vi "显示UI.vi"() -> ()   [LabVIEW 2016, in "国弘多参数.lvlib"]
uses:
  <vilib>/Utility/miscctls.llb/LVPointTypeDef.ctl
  <vilib>/Utility/config.llb/NI_LVConfig.lvlib
panel:
  out "运行状态":u16(ring) items=["空闲", "水样测试", "标样核查"]
  in  "叶绿素a校准":bool
  in  "停止":bool
  in  "标样核查":bool
  in  "水样测试":bool
  in  "关闭":bool
  in  "open MB":bool
  in  "设置":bool
  in  "水温校准":bool
  in  "浊度校准":bool
  in  "溶解氧校准":bool
  in  "电导率校准":bool
  in  "pH校准":bool
  in  "探头校正返回":bool
  in  "探头校正":bool
  in  "浊度参数查询":bool
  in  "溶解氧参数查询":bool
  in  "电导率参数查询":bool
  in  "pH参数查询":bool
  out "检测值":T1
  in  "返回":bool
  in  "参数查询":bool
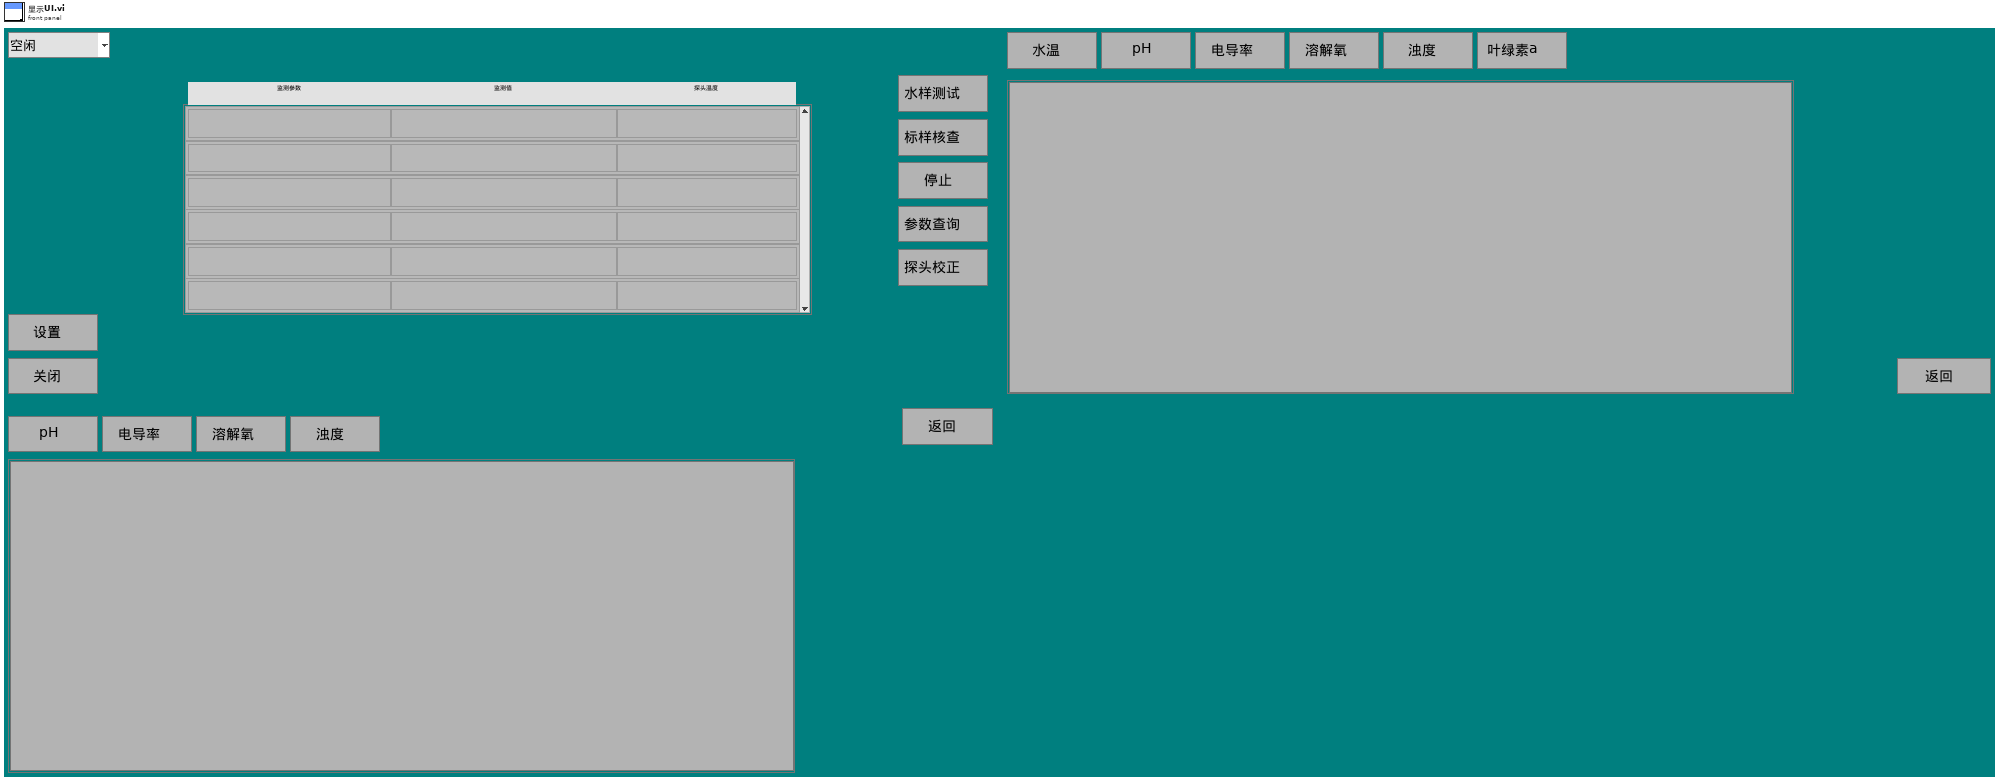
[diagram p1: front panel]
types:
  T1 = typedef "国弘多参数.lvlib/检测值.ctl" = cluster{"监测参数1":string, "浓度1":string, "探头温度1":string}[]
  T2 = typedef "LVPointTypeDef.ctl" = cluster{"Horizontal":i16, "Vertical":i16}
  T3 = cluster{"电极状态标志":u16, "电极型号标志":u16, "溶解氧测量值":sgl, "温度测量值":sgl, "溶解氧饱和度值":sgl, "盐度补偿值":sgl, "大气压补偿值":sgl, "溶解氧偏移修正值":sgl, "温度偏移修正值":sgl, "手动温度补偿值":sgl, "溶解氧电极零点":sgl, "溶解氧电极斜率":sgl, "第1点标准值记录":sgl, "第1点信号值记录":sgl, "第1点温度值记录":sgl, "第2点标准值记录":sgl, "第2点信号值记录":sgl, "第2点温度值记录":sgl, "命令滤波设定":u16, "温度模式":enum16{"ATC", "MTC"}, "生产批次":u16, "电极序号":u16, "串口地址":u16, "串口波特率":enum16{"9600", "19200", "115200"}, "串口校验位":enum16{"NONE", "ODD", "EVEN"}, "串口停止位":enum16{"1bit", "2bit"}, "第一点标准值":sgl, "第二点标准值":sgl}
  T4 = cluster{"电极状态标志":u16, "电极型号标志":u16, "酸碱度测量值":sgl, "温度测量值":sgl, "酸碱度信号值":sgl, "温度信号值":sgl, "酸碱度偏移修正值":sgl, "温度偏移修正值":sgl, "手动温度补偿值":sgl, "酸碱度电极零点":sgl, "酸碱度电极斜率":sgl, "第1点标准值记录":sgl, "第1点信号值记录":sgl, "第1点温度值记录":sgl, "第2点标准值记录":sgl, "第2点信号值记录":sgl, "第2点温度值记录":sgl, "命令滤波设定":u16, "温度模式":enum16{"ATC", "MTC"}, "生产批次":u16, "电极序号":u16, "串口地址":u16, "串口波特率":enum16{"9600", "19200", "115200"}, "串口校验位":enum16{"NONE", "ODD", "EVEN"}, "串口停止位":enum16{"1bit", "2bit"}, "第一点标准值":sgl, "第二点标准值":sgl}
  T5 = cluster{"电极状态标志":u16, "电极型号标志":u16, "浊度测量值":sgl, "温度测量值":sgl, "浊度信号值":sgl, "浊度偏移修正值":sgl, "温度偏移修正值":sgl, "手动温度补偿值":sgl, "浊度电极零点":sgl, "浊度电极斜率":sgl, "第1点标准值记录":sgl, "第1点信号值记录":sgl, "第1点温度值记录":sgl, "第2点标准值记录":sgl, "第2点信号值记录":sgl, "第2点温度值记录":sgl, "命令滤波设定":u16, "温度模式":enum16{"ATC", "MTC"}, "生产批次":u16, "电极序号":u16, "串口地址":u16, "串口波特率":enum16{"9600", "19200", "115200"}, "串口校验位":enum16{"NONE", "ODD", "EVEN"}, "串口停止位":enum16{"1bit", "2bit"}, "第一点标准值":sgl, "第二点标准值":sgl}
  T6 = cluster{"电极状态标志":u16, "电极型号标志":u16, "电导率测量值":sgl, "温度测量值":sgl, "电导率信号值":sgl, "温度信号值":sgl, "温度补偿系数":sgl, "电导率偏移修正值":sgl, "温度偏移修正值":sgl, "手动温度补偿值":sgl, "电导率电极零点":sgl, "电导率电极斜率":sgl, "命令滤波设定":u16, "温度模式":enum16{"ATC", "MTC"}, "生产批次":u16, "电极序号":u16, "串口地址":u16, "串口波特率":enum16{"9600", "19200", "115200"}, "串口校验位":enum16{"NONE", "ODD", "EVEN"}, "串口停止位":enum16{"1bit", "2bit"}, "第一点标准值":sgl, "第二点标准值":sgl}
  T7 = cluster{"监测参数1":string, "浓度1":string, "探头温度1":string}[]
  T8 = cluster{"CH":u16, "监测值":dbl, "监测信号值":dbl, "温度偏移修正值":sgl}
  T9 = typedef "NI_LVConfig.lvlib/Config Data RefNum.ctl" = refnum<k1>
  T10 = cluster{"baud rate (bps)":u32, "stop bits":u16, "parity":u16, "flow control":u16, "timeout":u32, "retries":i32}
  T11 = enum32{"Bad", "Idle", "Run top level", "Running"}
  T12 = cluster{"数据保存间隔":dbl, "水温标样值":dbl, "pH标样值":dbl, "溶解氧标样值":dbl, "电导率标样值":dbl, "浊度标样值":dbl}
  T13 = cluster{"Temp":bool, "pH":bool, "DO":bool, "Cond":bool, "Turb":bool, "叶绿素a启用":bool}
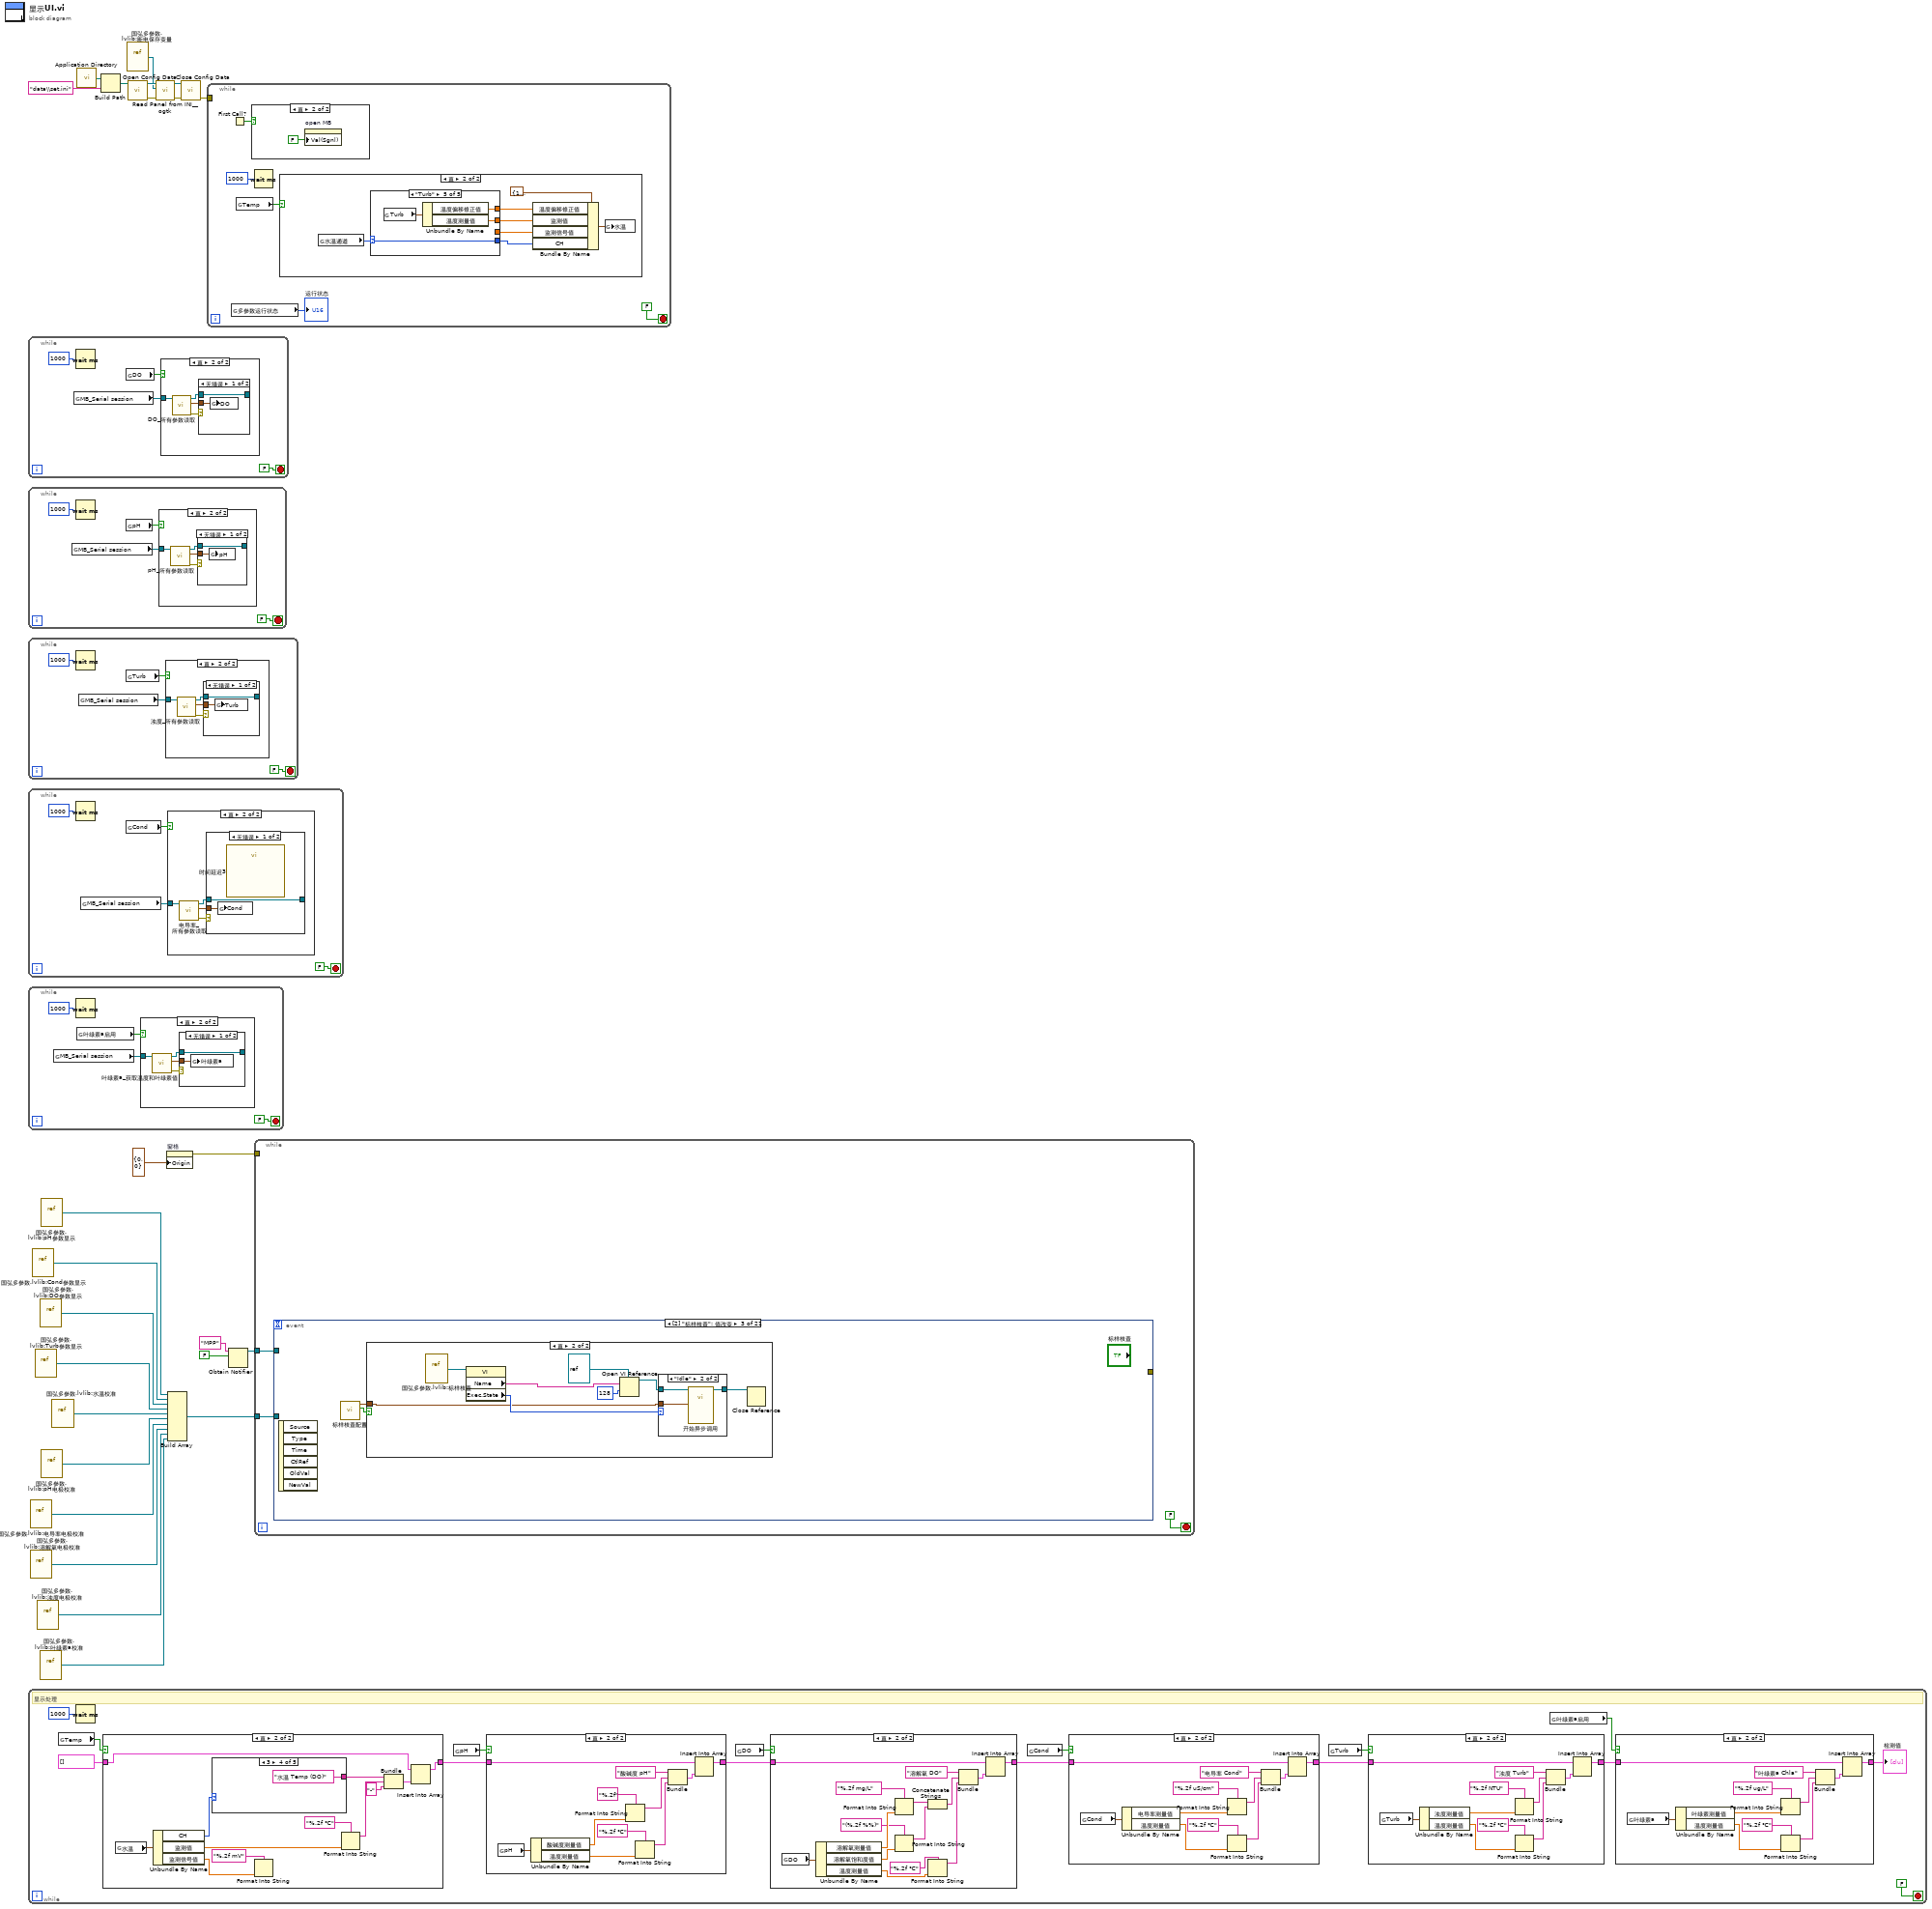
[diagram p0: block diagram]
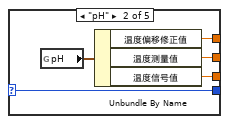
[diagram p14: hidden frame]
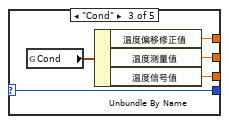
[diagram p15: hidden frame]
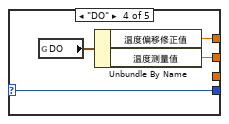
[diagram p16: hidden frame]
diagram:
  n1 = while {
    stop <- FALSE stop-if-true
    n2 = global read "过程全局变量.vi" "MB_Serial session"() -> (w26:refnum<class "MB_Master_Serial.lvclass">)
    n3 = Wait (ms)(milliseconds to wait=u32 1000 ("等待时间（毫秒）")) -> ()  [unwired: 1 out]
    n4 = global read "断电保存变量.vi" "DO"() -> (w27:bool)
    n5 = case shown="真" w27 {
      tunnel: w26 -> [_ w30]
      frame False {
      }
      frame True {
        n6 = call "DO_所有参数读取.vi"("MB_Serial session in"=w30) -> ("error out"=w32:errorcluster, "输出值"=w33:T3, "MB_Serial session out"=w31:refnum<class "MB_Master_Serial.lvclass">)  [unwired: 8 in]
        n7 = case shown="无错误" w32 {
          tunnel: w33 -> [w35 _]
          tunnel: w31 -> [w34 w36]
          tunnel: [w34 w36] -> _
          frame No Error {
            n8 = global write "过程全局变量.vi" "DO"(w35) -> ()
          }
          frame Error {
          }
        }
      }
    }
  }
  n9 = while {
    stop <- FALSE stop-if-true
    n10 = global read "过程全局变量.vi" "MB_Serial session"() -> (w38:refnum<class "MB_Master_Serial.lvclass">)
    n11 = Wait (ms)(milliseconds to wait=u32 1000 ("等待时间（毫秒）")) -> ()  [unwired: 1 out]
    n12 = global read "断电保存变量.vi" "pH"() -> (w39:bool)
    n13 = case shown="真" w39 {
      tunnel: w38 -> [_ w41]
      frame False {
      }
      frame True {
        n14 = call "pH_所有参数读取.vi"("MB_Serial session in"=w41) -> ("error out"=w43:errorcluster, "输出值"=w44:T4, "MB_Serial session out"=w42:refnum<class "MB_Master_Serial.lvclass">)  [unwired: 8 in]
        n15 = case shown="无错误" w43 {
          tunnel: w44 -> [w46 _]
          tunnel: w42 -> [w45 w47]
          tunnel: [w45 w47] -> _
          frame No Error {
            n16 = global write "过程全局变量.vi" "pH"(w46) -> ()
          }
          frame Error {
          }
        }
      }
    }
  }
  n17 = while {
    stop <- FALSE stop-if-true
    n18 = Wait (ms)(milliseconds to wait=u32 1000 ("等待时间（毫秒）")) -> ()  [unwired: 1 out]
    n19 = global read "过程全局变量.vi" "MB_Serial session"() -> (w49:refnum<class "MB_Master_Serial.lvclass">)
    n20 = global read "断电保存变量.vi" "Turb"() -> (w50:bool)
    n21 = case shown="真" w50 {
      tunnel: w49 -> [_ w52]
      frame False {
      }
      frame True {
        n22 = call "浊度_所有参数读取.vi"("MB_Serial session in"=w52) -> ("error out"=w54:errorcluster, "输出值"=w55:T5, "MB_Serial session out"=w53:refnum<class "MB_Master_Serial.lvclass">)  [unwired: 8 in]
        n23 = case shown="无错误" w54 {
          tunnel: w55 -> [w57 _]
          tunnel: w53 -> [w56 w58]
          tunnel: [w56 w58] -> _
          frame No Error {
            n24 = global write "过程全局变量.vi" "Turb"(w57) -> ()
          }
          frame Error {
          }
        }
      }
    }
  }
  n25 = while {
    stop <- FALSE stop-if-true
    n26 = Wait (ms)(milliseconds to wait=u32 1000 ("等待时间（毫秒）")) -> ()  [unwired: 1 out]
    n27 = global read "过程全局变量.vi" "MB_Serial session"() -> (w60:refnum<class "MB_Master_Serial.lvclass">)
    n28 = global read "断电保存变量.vi" "Cond"() -> (w61:bool)
    n29 = case shown="真" w61 {
      tunnel: w60 -> [_ w63]
      frame False {
      }
      frame True {
        n30 = call "电导率_所有参数读取.vi"("MB_Serial session in"=w63) -> ("error out"=w65:errorcluster, "输出值"=w66:T6, "MB_Serial session out"=w64:refnum<class "MB_Master_Serial.lvclass">)  [unwired: 8 in]
        n31 = case shown="无错误" w65 {
          tunnel: w66 -> [w68 _]
          tunnel: [w67 w69] -> _
          tunnel: w64 -> [w67 w69]
          frame No Error {
            n32 = global write "过程全局变量.vi" "Cond"(w68) -> ()
            n33 = call "时间延迟3"() -> ()  [unwired: 11 in, 1 out]
          }
          frame Error {
          }
        }
      }
    }
  }
  n34 = while {
    stop <- FALSE stop-if-true
    n35 = global read "过程全局变量.vi" "MB_Serial session"() -> (w72:refnum<class "MB_Master_Serial.lvclass">)
    n36 = Wait (ms)(milliseconds to wait=u32 1000 ("等待时间（毫秒）")) -> ()  [unwired: 1 out]
    n37 = global read "断电保存变量.vi" "叶绿素a启用"() -> (w71:bool)
    n38 = case shown="真" w71 {
      tunnel: w72 -> [_ w74]
      frame False {
      }
      frame True {
        n39 = call "叶绿素a_获取温度和叶绿素值.vi"("MB_Serial session in"=w74) -> ("error out"=w76:errorcluster, "输出值"=w77:cluster{"温度测量值":sgl, "叶绿素测量值":sgl, "错误标志":u16}, "MB_Serial session out"=w75:refnum<class "MB_Master_Serial.lvclass">)  [unwired: 8 in]
        n40 = case shown="无错误" w76 {
          tunnel: w77 -> [w79 _]
          tunnel: w75 -> [w78 w80]
          tunnel: [w78 w80] -> _
          frame No Error {
            n41 = global write "过程全局变量.vi" "叶绿素a"(w79) -> ()
          }
          frame Error {
          }
        }
      }
    }
  }
  n42 = while {
    stop <- FALSE stop-if-true
    # "显示处理"
    n43 = global read "断电保存变量.vi" "Temp"() -> (w93:bool)
    n44 = Wait (ms)(milliseconds to wait=u32 1000 ("等待时间（毫秒）")) -> ()  [unwired: 1 out]
    n45 = case shown="真" w93 {
      tunnel: [w160 w161] -> w90
      tunnel: T7 [] ("数组") -> [w160 w162]
      frame False {
      }
      frame True {
        n46 = global read "过程全局变量.vi" "水温"() -> (w172:T8)
        n47 = Unbundle By Name(w172) -> ("CH"=w167:u16, "监测值"=w170:dbl, "监测信号值"=w168:dbl)
        n48 = case shown="3" w167 {
          tunnel: ["水温 Temp" ("监测参数1") "水温 Temp (pH)" ("监测参数1") "水温 Temp (Cond)" ("监测参数1") "水温 Temp (DO)" ("监测参数1") "水温 Temp (Turb)" ("监测参数1")] -> w166
          frame 0, Default {
          }
          frame 1 {
          }
          frame 2 {
          }
          frame 3 {
          }
          frame 4 {
          }
        }
        n49 = Format Into String(format string="%.2f mV" ("格式字符串"), w168) -> ()  [unwired: 2 in, 2 out]
        n50 = Format Into String(format string="%.2f ℃" ("格式字符串"), w170) -> (resulting string=w165:string)  [unwired: 2 in, 1 out]
        n51 = Bundle("监测参数1"=w166, w165, "探头温度1"="-") -> (w163:cluster{"监测参数1":string, string, "探头温度1":string})  [unwired: 1 in]
        n52 = Insert Into Array(array=w162, new element=w163) -> (w161:T7)  [unwired: 1 in]
      }
    }
    n53 = global read "断电保存变量.vi" "pH"() -> (w91:bool)
    n54 = case shown="真" w91 {
      tunnel: [w148 w149] -> w88
      tunnel: w90 -> [w148 w151]
      frame False {
      }
      frame True {
        n55 = global read "过程全局变量.vi" "pH"() -> (w159:T4)
        n56 = Unbundle By Name(w159) -> ("酸碱度测量值"=w158:sgl, "温度测量值"=w156:sgl)
        n57 = Format Into String(format string="%.2f" ("格式字符串"), w158) -> (resulting string=w152:string)  [unwired: 2 in, 1 out]
        n58 = Format Into String(format string="%.2f ℃" ("格式字符串"), w156) -> (resulting string=w154:string)  [unwired: 2 in, 1 out]
        n59 = Bundle("监测参数2"="酸碱度 pH", w152, w154) -> (w150:cluster{"监测参数2":string, string, string})  [unwired: 1 in]
        n60 = Insert Into Array(array=w151, new element=w150) -> (w149:T7)  [unwired: 1 in]
      }
    }
    n61 = global read "断电保存变量.vi" "DO"() -> (w89:bool)
    n62 = case shown="真" w89 {
      tunnel: [w132 w133] -> w85
      tunnel: w88 -> [w132 w134]
      frame False {
      }
      frame True {
        n63 = global read "过程全局变量.vi" "DO"() -> (w143:T3)
        n64 = Unbundle By Name(w143) -> ("溶解氧测量值"=w144:sgl, "溶解氧饱和度值"=w141:sgl, "温度测量值"=w146:sgl)
        n65 = Format Into String(format string="%.2f mg/L" ("格式字符串"), w144) -> (resulting string=w140:string)  [unwired: 2 in, 1 out]
        n66 = Format Into String(format string="(%.2f %%)" ("格式字符串"), w141) -> (resulting string=w139:string)  [unwired: 2 in, 1 out]
        n67 = Concatenate Strings(w140, w139) -> (w138:string)
        n68 = Format Into String(format string="%.2f ℃" ("格式字符串"), w146) -> (resulting string=w136:string)  [unwired: 2 in, 1 out]
        n69 = Bundle("监测参数2"="溶解氧 DO", w138, w136) -> (w135:cluster{"监测参数2":string, string, string})  [unwired: 1 in]
        n70 = Insert Into Array(array=w134, new element=w135) -> (w133:T7)  [unwired: 1 in]
      }
    }
    n71 = global read "断电保存变量.vi" "Cond"() -> (w87:bool)
    n72 = case shown="真" w87 {
      tunnel: w85 -> [w120 w123]
      tunnel: [w120 w121] -> w84
      frame False {
      }
      frame True {
        n73 = global read "过程全局变量.vi" "Cond"() -> (w131:T6)
        n74 = Unbundle By Name(w131) -> ("电导率测量值"=w130:sgl, "温度测量值"=w128:sgl)
        n75 = Format Into String(format string="%.2f uS/cm" ("格式字符串"), w130) -> (resulting string=w124:string)  [unwired: 2 in, 1 out]
        n76 = Format Into String(format string="%.2f ℃" ("格式字符串"), w128) -> (resulting string=w125:string)  [unwired: 2 in, 1 out]
        n77 = Bundle("监测参数2"="电导率 Cond", w124, w125) -> (w122:cluster{"监测参数2":string, string, string})  [unwired: 1 in]
        n78 = Insert Into Array(array=w123, new element=w122) -> (w121:T7)  [unwired: 1 in]
      }
    }
    n79 = global read "断电保存变量.vi" "Turb"() -> (w86:bool)
    n80 = case shown="真" w86 {
      tunnel: w84 -> [w108 w111]
      tunnel: [w108 w109] -> w83
      frame False {
      }
      frame True {
        n81 = global read "过程全局变量.vi" "Turb"() -> (w115:T5)
        n82 = Unbundle By Name(w115) -> ("浊度测量值"=w116:sgl, "温度测量值"=w118:sgl)
        n83 = Format Into String(format string="%.2f NTU" ("格式字符串"), w116) -> (resulting string=w113:string)  [unwired: 2 in, 1 out]
        n84 = Format Into String(format string="%.2f ℃" ("格式字符串"), w118) -> (resulting string=w114:string)  [unwired: 2 in, 1 out]
        n85 = Bundle("监测参数2"="浊度 Turb", w113, w114) -> (w110:cluster{"监测参数2":string, string, string})  [unwired: 1 in]
        n86 = Insert Into Array(array=w111, new element=w110) -> (w109:T7)  [unwired: 1 in]
      }
    }
    n87 = global read "断电保存变量.vi" "叶绿素a启用"() -> (w81:bool)
    n88 = case shown="真" w81 {
      tunnel: w83 -> [w96 w99]
      tunnel: [w96 w97] -> w82
      frame False {
      }
      frame True {
        n89 = global read "过程全局变量.vi" "叶绿素a"() -> (w103:cluster{"温度测量值":sgl, "叶绿素测量值":sgl, "错误标志":u16})
        n90 = Unbundle By Name(w103) -> ("叶绿素测量值"=w104:sgl, "温度测量值"=w106:sgl)
        n91 = Format Into String(format string="%.2f ug/L" ("格式字符串"), w104) -> (resulting string=w101:string)  [unwired: 2 in, 1 out]
        n92 = Format Into String(format string="%.2f ℃" ("格式字符串"), w106) -> (resulting string=w102:string)  [unwired: 2 in, 1 out]
        n93 = Bundle("监测参数2"="叶绿素a Chla", w101, w102) -> (w98:cluster{"监测参数2":string, string, string})  [unwired: 1 in]
        n94 = Insert Into Array(array=w99, new element=w98) -> (w97:T7)  [unwired: 1 in]
      }
    }
    "检测值" <- w82
  }
  n95 = vi-ref "国弘多参数.lvlib:电导率电极校准.vi"() -> (w16:refnum<vi>)
  n96 = vi-ref "国弘多参数.lvlib:溶解氧电极校准.vi"() -> (w15:refnum<vi>)
  n97 = vi-ref "国弘多参数.lvlib:Cond参数显示.vi"() -> (w22:refnum<vi>)
  n98 = vi-ref "国弘多参数.lvlib:Turb参数显示.vi"() -> (w20:refnum<vi>)
  n99 = vi-ref "国弘多参数.lvlib:浊度电极校准.vi"() -> (w14:refnum<vi>)
  n100 = vi-ref "国弘多参数.lvlib:DO参数显示.vi"() -> (w21:refnum<vi>)
  n101 = vi-ref "国弘多参数.lvlib:叶绿素a校准.vi"() -> (w4:refnum<vi>)
  n102 = vi-ref "国弘多参数.lvlib:pH参数显示.vi"() -> (w23:refnum<vi>)
  n103 = vi-ref "国弘多参数.lvlib:pH电极校准.vi"() -> (w17:refnum<vi>)
  n104 = vi-ref "国弘多参数.lvlib:水温校准.vi"() -> (w18:refnum<vi>)
  n105 = call <vilib>:"Application Directory.vi"() -> ("Application Directory"=w9:path)
  n106 = Build Path(base path=w9, name or relative path="data\\set.ini" ("名称或相对路径")) -> (appended path=w8:path)
  n107 = vi-ref "国弘多参数.lvlib:断电保存变量.vi"() -> (w6:refnum<vi>)
  n108 = call <vilib>:"Open Config Data.vi"("configuration file path"=w8) -> ("error out"=w12:errorcluster, "refnum"=w13:T9)  [unwired: 8 in, 1 out]
  n109 = call <userlib>:"Read Panel from INI__ogtk.vi"("error in (no error)"=w12, "VI ref"=w6, "refnum"=w13) -> ("error out"=w10:errorcluster, "refnum out"=w11:T9)  [unwired: 7 in]
  n110 = property on="窗格" class="Pane"("Origin"=T2 {"Horizontal"=0, "Vertical"=0} ("原点")) -> (error out=w25:errorcluster)  [unwired: 2 in, 1 out]
  n111 = Build Array(w23, w22, w21, w20, w18, w17, w16, w15, w14, w4) -> (w19:refnum<vi>[])
  n112 = call <vilib>:"Close Config Data.vi"("error in (no error)"=w10, "refnum"=w11) -> ("error out"=w5:errorcluster)  [unwired: 8 in, 1 out]
  n113 = while {
    tunnel: w5 -> [_]
    stop <- FALSE stop-if-true
    n114 = First Call?() -> (First Call?: T/F=w180:bool)
    n115 = global read "过程全局变量.vi" "多参数运行状态"() -> (→"运行状态":u16)
    n116 = global read "断电保存变量.vi" "Temp"() -> (w179:bool)
    n117 = case shown="真" w180 {
      frame False {
      }
      frame True {
        n118 = property on="open MB" class="Bool (严格)"("Val(Sgnl)"=FALSE ("值(信号)")) -> ()  [unwired: 2 in, 2 out]
      }
    }
    n119 = Wait (ms)(milliseconds to wait=u32 1000 ("等待时间（毫秒）")) -> ()  [unwired: 1 out]
    n120 = case shown="真" w179 {
      frame False {
      }
      frame True {
        n121 = global read "断电保存变量.vi" "水温通道"() -> (w189:enum16{"NULL", "pH", "Cond", "DO", "Turb"})
        n122 = case shown="\"Turb\"" w189 {
          selector: w189 -> [w190 w195 w200 w204 w208]
          tunnel: [w190 w195 w200 w204 w208] -> w188
          tunnel: [_ w193 w198 w202 w206] -> w187
          tunnel: [_ w192 w197 _ _] -> w186
          tunnel: [_ w191 w196 w201 w205] -> w183
          frame "NULL", Default {
          }
          frame "pH" {
            n123 = global read "过程全局变量.vi" "pH"() -> (w194:T4)
            n124 = Unbundle By Name(w194) -> ("温度偏移修正值"=w191:sgl, "温度测量值"=w193:sgl, "温度信号值"=w192:sgl)
          }
          frame "Cond" {
            n125 = global read "过程全局变量.vi" "Cond"() -> (w199:T6)
            n126 = Unbundle By Name(w199) -> ("温度偏移修正值"=w196:sgl, "温度测量值"=w198:sgl, "温度信号值"=w197:sgl)
          }
          frame "DO" {
            n127 = global read "过程全局变量.vi" "DO"() -> (w203:T3)
            n128 = Unbundle By Name(w203) -> ("温度偏移修正值"=w201:sgl, "温度测量值"=w202:sgl)
          }
          frame "Turb" {
            n129 = global read "过程全局变量.vi" "Turb"() -> (w207:T5)
            n130 = Unbundle By Name(w207) -> ("温度偏移修正值"=w205:sgl, "温度测量值"=w206:sgl)
          }
        }
        n131 = Bundle By Name(cluster=T8 {"CH"=1, "监测值"=0.0, "监测信号值"=0.0, "温度偏移修正值"=0.0} ("水温"), "温度偏移修正值"=w183, "监测值"=w187, "监测信号值"=w186, "CH"=w188) -> (w185:T8)
        n132 = global write "过程全局变量.vi" "水温"(w185) -> ()
      }
    }
  }
  n133 = Obtain Notifier(name (unnamed)="MPP" ("名称（未命名）"), notification data type=FALSE) -> (notifier out=w1:refnum<notifier>)  [unwired: 2 in, 2 out]
  n134 = while {
    tunnel: w25 -> [_]
    tunnel: w19 -> [w211]
    tunnel: w1 -> [w210]
    stop <- FALSE stop-if-true
    n135 = event shown="[2] \"标样核查\": 值改变" {
      selector: _ -> [_ _ _ _ _ _ _ _ _ _ _ _ _ _ _ _ _ _ _ _ _]
      dyn-events: _ -> [_ _ _ _ _ _ _ _ _ _ _ _ _ _ _ _ _ _ _ _ _]
      timeout: _ -> [_ _ _ _ _ _ _ _ _ _ _ _ _ _ _ _ _ _ _ _ _]
      tunnel: w211 -> [_ _ _ _ _ _ _ w275 w287 w299 w307 w318 w330 w342 w354 w366 w378 w390 w402 w414 w426]
      tunnel: [_ _ _ _ _ w247 _ _ _ _ _ _ _ _ _ _ _ _ _ _ _] -> _
      tunnel: w210 -> [_ _ _ w244 _ _ _ _ _ _ _ _ _ _ _ _ _ _ _ _ _]
      event Timeout {
        n136 = event-data() -> ()  [unwired: 1 in, 3 out]
      }
      event "水样测试": Value Change {
        n137 = event-data() -> ()  [unwired: 1 in, 6 out]
        n138 = call "水样测试配置.vi"() -> ("确认输出"=w214:bool, "水样测定时间输出"=w213:dbl)  [unwired: 10 in]
        n139 = case shown="真" w214 {
          tunnel: w213 -> [_ w217]
          frame False {
          }
          frame True {
            n140 = vi-ref "国弘多参数.lvlib:水样测试.vi"() -> (w218:refnum<vi>)
            n141 = property class="VI"(reference=w218) -> ("Name"=w222:string, "Exec.State"=w220:T11)  [unwired: 1 in, 2 out]
            n142 = Open VI Reference(type specifier VI Refnum (for type only)=refnum<vi> refnum, vi path=w222, options=128 ("选项")) -> (vi reference=w223:refnum<vi>)  [unwired: 3 in, 1 out]
            n143 = case shown="\"Idle\"" w220 {
              tunnel: [w224 w228] -> w219
              tunnel: w223 -> [w224 w227]
              tunnel: w217 -> [_ w226]
              tunnel: "hd" ("数据标记表") -> [_ w225]
              frame "Bad", Default {
              }
              frame "Idle" {
                n144 = call-by-ref "开始异步调用"(reference=w227, "数据标记表"=w225, "水样测试时间"=w226) -> (reference out=w228:refnum<vi>)  [unwired: 11 in, 1 out]
              }
            }
            n145 = Close Reference(reference=w219) -> ()  [unwired: 1 in, 1 out]
          }
        }
      }
      event "标样核查": Value Change {
        n146 = event-data() -> ()  [unwired: 1 in, 6 out]
        n147 = call "标样核查配置.vi"() -> ("确认输出"=w230:bool, "标样核查配置"=w229:T12)  [unwired: 10 in]
        n148 = case shown="真" w230 {
          tunnel: w229 -> [_ w231]
          frame False {
          }
          frame True {
            n149 = vi-ref "国弘多参数.lvlib:标样核查.vi"() -> (w232:refnum<vi>)
            n150 = property class="VI"(reference=w232) -> ("Name"=w237:string, "Exec.State"=w234:T11)  [unwired: 1 in, 2 out]
            n151 = Open VI Reference(type specifier VI Refnum (for type only)=refnum<vi> refnum, vi path=w237, options=128 ("选项")) -> (vi reference=w238:refnum<vi>)  [unwired: 3 in, 1 out]
            n152 = case shown="\"Idle\"" w234 {
              tunnel: [w239 w242] -> w233
              tunnel: w238 -> [w239 w241]
              tunnel: w231 -> [_ w240]
              frame "Bad", Default {
              }
              frame "Idle" {
                n153 = call-by-ref "开始异步调用"(reference=w241, "标样核查配置"=w240) -> (reference out=w242:refnum<vi>)  [unwired: 12 in, 1 out]
              }
            }
            n154 = Close Reference(reference=w233) -> ()  [unwired: 1 in, 1 out]
          }
        }
      }
      event "停止": Value Change {
        n155 = event-data() -> ()  [unwired: 1 in, 6 out]
        n156 = Send Notification(notification=TRUE ("通知"), notifier=w244) -> ()  [unwired: 1 in, 2 out]
      }
      event "关闭": Value Change {
        n157 = event-data() -> ()  [unwired: 1 in, 6 out]
        n158 = flat-sequence {
          frame #0 {
            n159 = global read "过程全局变量.vi" "MB_Serial session"() -> (w245:refnum<class "MB_Master_Serial.lvclass">)
            n160 = call "close MB.vi"("MB_Serial session"=w245) -> ()  [unwired: 10 in, 1 out]
          }
          frame #1 {
            n161 = Quit LabVIEW() -> ()  [unwired: 1 in]
          }
        }
      }
      event "open MB": Value Change {
        n162 = event-data() -> ()  [unwired: 1 in, 6 out]
        n163 = global read "过程全局变量.vi" "MB_Serial session"() -> (w246:refnum<class "MB_Master_Serial.lvclass">)
        n164 = global read "断电保存变量.vi" "VISA资源名称"() -> (w250:refnum<visa-resource-name>)
        n165 = call "close MB.vi"("MB_Serial session"=w246) -> ("error out"=w248:errorcluster)  [unwired: 10 in]
        n166 = call "open MB.vi"("error in (no error)"=w248, "Serial Config"=T10 {"baud rate (bps)"=9600, "stop bits"=10, "parity"=0, "flow control"=0, "timeout"=1000, "retries"=1}, "VISA资源名称"=w250) -> ("error out"=w247:errorcluster, "MB_Serial session"=w249:refnum<class "MB_Master_Serial.lvclass">)  [unwired: 7 in]
        n167 = global write "过程全局变量.vi" "MB_Serial session"(w249) -> ()
      }
      event "设置": Value Change {
        n168 = event-data() -> ()  [unwired: 1 in, 6 out]
        n169 = flat-sequence {
          frame #0 {
            n170 = call "配置.vi"() -> ("启用参数"=w258:T13, "串口输出"=w259:refnum<visa-resource-name>)  [unwired: 10 in]
            n171 = global write "断电保存变量.vi" "VISA资源名称"(w259) -> ()
            n172 = Unbundle By Name(w258) -> ("Temp"=w253:bool, "pH"=w254:bool, "DO"=w255:bool, "Cond"=w256:bool, "Turb"=w257:bool, "叶绿素a启用"=w252:bool)
            n173 = global write "断电保存变量.vi" "pH"(w254) -> ()
            n174 = global write "断电保存变量.vi" "DO"(w255) -> ()
            n175 = global write "断电保存变量.vi" "Cond"(w256) -> ()
            n176 = global write "断电保存变量.vi" "Turb"(w257) -> ()
            n177 = global write "断电保存变量.vi" "Temp"(w253) -> ()
            n178 = global write "断电保存变量.vi" "叶绿素a启用"(w252) -> ()
          }
          frame #1 {
            n179 = call <vilib>:"Application Directory.vi"() -> ("Application Directory"=w269:path)
            n180 = Build Path(base path=w269, name or relative path="data\\set.ini" ("名称或相对路径")) -> (appended path=w268:path)
            n181 = call <vilib>:"Open Config Data.vi"("configuration file path"=w268) -> ("error out"=w272:errorcluster, "refnum"=w273:T9)  [unwired: 8 in, 1 out]
            n182 = vi-ref "国弘多参数.lvlib:断电保存变量.vi"() -> (w266:refnum<vi>)
            n183 = call <userlib>:"Write Panel to INI__ogtk.vi"("error in (no error)"=w272, "VI ref"=w266, "refnum"=w273) -> ("error out"=w270:errorcluster, "refnum out"=w271:T9)  [unwired: 7 in]
            n184 = call <vilib>:"Close Config Data.vi"("error in (no error)"=w270, "refnum"=w271) -> ("error out"=w262:errorcluster, "file path"=w263:path)  [unwired: 8 in]
            n185 = Open/Create/Replace File(file path (use dialog)=w263, error in=w262) -> (refnum out=w264:refnum<file>, error out=w265:errorcluster)  [unwired: 4 in, 1 out]
            n186 = Flush File(refnum=w264, error in=w265) -> (refnum out=w260:refnum<file>, error out=w261:errorcluster)
            n187 = Close File(refnum=w260, error in=w261) -> ()  [unwired: 2 out]
          }
          frame #2 {
            n188 = property on="open MB" class="Bool (严格)"("Val(Sgnl)"=FALSE ("值(信号)")) -> ()  [unwired: 2 in, 2 out]
          }
        }
      }
      event "探头校正返回": Value Change {
        n189 = event-data() -> ()  [unwired: 1 in, 6 out]
        n190 = property on="窗格" class="Pane"("Origin"=T2 {"Horizontal"=0, "Vertical"=0} ("原点")) -> ()  [unwired: 2 in, 2 out]
        n191 = for {
          tunnel: w275 -> [w279] mode=indexing
          n192 = property class="VI"(reference=w279) -> (reference out=w277:refnum<vi>, "Exec.State"=w278:T11)  [unwired: 1 in, 1 out]
          n193 = case shown="\"Run top level\"" w278 {
            tunnel: w277 -> [_ _ w280 w281]
            frame "Bad", Default {
            }
            frame "Idle" {
            }
            frame "Run top level" {
              n194 = invoke class="VI" method="Abort VI"(reference=w280) -> ()  [unwired: 2 in, 3 out]
            }
            frame "Running" {
              n195 = invoke class="VI" method="Abort VI"(reference=w281) -> ()  [unwired: 2 in, 3 out]
            }
          }
        }
      }
      event "探头校正": Value Change {
        n196 = event-data() -> ()  [unwired: 1 in, 6 out]
        n197 = property on="窗格" class="Pane"("Origin"=T2 {"Horizontal"=1656, "Vertical"=0} ("原点")) -> ()  [unwired: 2 in, 2 out]
        n198 = Index Array(array=w287, index=4 ("索引")) -> (element=w288:refnum<vi>)
        n199 = property class="VI"(reference=w288) -> (reference out=w283:refnum<vi>, "Exec.State"=w282:T11)  [unwired: 1 in, 1 out]
        n200 = case shown="\"Bad\", 默认" w282 {
          tunnel: [w290 w292] -> w286
          tunnel: w283 -> [w290 w291]
          frame "Bad", Default {
          }
          frame "Idle" {
            n201 = invoke class="VI" method="Run VI"(reference=w291, "Wait until done"=FALSE ("结束前等待"), "Auto Dispose Ref"=FALSE ("自动销毁引用")) -> (reference out=w292:refnum<vi>)  [unwired: 2 in, 4 out]
          }
        }
        n202 = invoke on="探头校准子面板" class="SubPnl" method="Remove VI"() -> (error out=w285:errorcluster)  [unwired: 3 in, 2 out]
        n203 = invoke on="探头校准子面板" class="SubPnl" method="Insert VI"(error in=w285, "VI Ref"=w286) -> ()  [unwired: 2 in, 4 out]
      }
      event "参数查询": Value Change {
        n204 = event-data() -> ()  [unwired: 1 in, 6 out]
        n205 = property on="窗格" class="Pane"("Origin"=T2 {"Horizontal"=0, "Vertical"=628} ("原点")) -> ()  [unwired: 2 in, 2 out]
        n206 = Index Array(array=w299) -> (element=w300:refnum<vi>)  [unwired: 1 in]
        n207 = property class="VI"(reference=w300) -> (reference out=w296:refnum<vi>, "Exec.State"=w295:T11)  [unwired: 1 in, 1 out]
        n208 = case shown="\"Bad\", 默认" w295 {
          tunnel: [w302 w304] -> w298
          tunnel: w296 -> [w302 w303]
          frame "Bad", Default {
          }
          frame "Idle" {
            n209 = invoke class="VI" method="Run VI"(reference=w303, "Wait until done"=FALSE ("结束前等待"), "Auto Dispose Ref"=FALSE ("自动销毁引用")) -> (reference out=w304:refnum<vi>)  [unwired: 2 in, 4 out]
          }
        }
        n210 = invoke on="参数查询子面板" class="SubPnl" method="Remove VI"() -> (error out=w297:errorcluster)  [unwired: 3 in, 2 out]
        n211 = invoke on="参数查询子面板" class="SubPnl" method="Insert VI"(error in=w297, "VI Ref"=w298) -> ()  [unwired: 2 in, 4 out]
      }
      event "返回": Value Change {
        n212 = event-data() -> ()  [unwired: 1 in, 6 out]
        n213 = property on="窗格" class="Pane"("Origin"=T2 {"Horizontal"=0, "Vertical"=0} ("原点")) -> ()  [unwired: 2 in, 2 out]
        n214 = for {
          tunnel: w307 -> [w311] mode=indexing
          n215 = property class="VI"(reference=w311) -> (reference out=w309:refnum<vi>, "Exec.State"=w310:T11)  [unwired: 1 in, 1 out]
          n216 = case shown="\"Run top level\"" w310 {
            tunnel: w309 -> [_ _ w312 w313]
            frame "Bad", Default {
            }
            frame "Idle" {
            }
            frame "Run top level" {
              n217 = invoke class="VI" method="Abort VI"(reference=w312) -> ()  [unwired: 2 in, 3 out]
            }
            frame "Running" {
              n218 = invoke class="VI" method="Abort VI"(reference=w313) -> ()  [unwired: 2 in, 3 out]
            }
          }
        }
      }
      event "pH参数查询": Value Change {
        n219 = event-data() -> ()  [unwired: 1 in, 6 out]
        n220 = Index Array(array=w318) -> (element=w319:refnum<vi>)  [unwired: 1 in]
        n221 = property class="VI"(reference=w319) -> (reference out=w315:refnum<vi>, "Exec.State"=w314:T11)  [unwired: 1 in, 1 out]
        n222 = case shown="\"Bad\", 默认" w314 {
          tunnel: [w320 w322] -> w317
          tunnel: w315 -> [w320 w321]
          frame "Bad", Default {
          }
          frame "Idle" {
            n223 = invoke class="VI" method="Run VI"(reference=w321, "Wait until done"=FALSE ("结束前等待"), "Auto Dispose Ref"=FALSE ("自动销毁引用")) -> (reference out=w322:refnum<vi>)  [unwired: 2 in, 4 out]
          }
        }
        n224 = invoke on="参数查询子面板" class="SubPnl" method="Remove VI"() -> (error out=w316:errorcluster)  [unwired: 3 in, 2 out]
        n225 = invoke on="参数查询子面板" class="SubPnl" method="Insert VI"(error in=w316, "VI Ref"=w317) -> ()  [unwired: 2 in, 4 out]
      }
      event "电导率参数查询": Value Change {
        n226 = event-data() -> ()  [unwired: 1 in, 6 out]
        n227 = Index Array(array=w330, index=1 ("索引")) -> (element=w331:refnum<vi>)
        n228 = property class="VI"(reference=w331) -> (reference out=w326:refnum<vi>, "Exec.State"=w325:T11)  [unwired: 1 in, 1 out]
        n229 = case shown="\"Bad\", 默认" w325 {
          tunnel: w326 -> [w332 w336]
          tunnel: [w332 w333] -> w328
          frame "Bad", Default {
          }
          frame "Idle" {
            n230 = invoke class="VI" method="Run VI"(reference=w336, "Wait until done"=FALSE ("结束前等待"), "Auto Dispose Ref"=FALSE ("自动销毁引用")) -> (reference out=w333:refnum<vi>)  [unwired: 2 in, 4 out]
          }
        }
        n231 = invoke on="参数查询子面板" class="SubPnl" method="Remove VI"() -> (error out=w327:errorcluster)  [unwired: 3 in, 2 out]
        n232 = invoke on="参数查询子面板" class="SubPnl" method="Insert VI"(error in=w327, "VI Ref"=w328) -> ()  [unwired: 2 in, 4 out]
      }
      event "溶解氧参数查询": Value Change {
        n233 = event-data() -> ()  [unwired: 1 in, 6 out]
        n234 = Index Array(array=w342, index=2 ("索引")) -> (element=w343:refnum<vi>)
        n235 = property class="VI"(reference=w343) -> (reference out=w338:refnum<vi>, "Exec.State"=w337:T11)  [unwired: 1 in, 1 out]
        n236 = case shown="\"Bad\", 默认" w337 {
          tunnel: [w344 w346] -> w340
          tunnel: w338 -> [w344 w345]
          frame "Bad", Default {
          }
          frame "Idle" {
            n237 = invoke class="VI" method="Run VI"(reference=w345, "Wait until done"=FALSE ("结束前等待"), "Auto Dispose Ref"=FALSE ("自动销毁引用")) -> (reference out=w346:refnum<vi>)  [unwired: 2 in, 4 out]
          }
        }
        n238 = invoke on="参数查询子面板" class="SubPnl" method="Remove VI"() -> (error out=w339:errorcluster)  [unwired: 3 in, 2 out]
        n239 = invoke on="参数查询子面板" class="SubPnl" method="Insert VI"(error in=w339, "VI Ref"=w340) -> ()  [unwired: 2 in, 4 out]
      }
      event "浊度参数查询": Value Change {
        n240 = event-data() -> ()  [unwired: 1 in, 6 out]
        n241 = Index Array(array=w354, index=3 ("索引")) -> (element=w355:refnum<vi>)
        n242 = property class="VI"(reference=w355) -> (reference out=w350:refnum<vi>, "Exec.State"=w349:T11)  [unwired: 1 in, 1 out]
        n243 = case shown="\"Bad\", 默认" w349 {
          tunnel: [w356 w358] -> w352
          tunnel: w350 -> [w356 w357]
          frame "Bad", Default {
          }
          frame "Idle" {
            n244 = invoke class="VI" method="Run VI"(reference=w357, "Wait until done"=FALSE ("结束前等待"), "Auto Dispose Ref"=FALSE ("自动销毁引用")) -> (reference out=w358:refnum<vi>)  [unwired: 2 in, 4 out]
          }
        }
        n245 = invoke on="参数查询子面板" class="SubPnl" method="Remove VI"() -> (error out=w351:errorcluster)  [unwired: 3 in, 2 out]
        n246 = invoke on="参数查询子面板" class="SubPnl" method="Insert VI"(error in=w351, "VI Ref"=w352) -> ()  [unwired: 2 in, 4 out]
      }
      event "水温校准": Value Change {
        n247 = event-data() -> ()  [unwired: 1 in, 6 out]
        n248 = Index Array(array=w366, index=4 ("索引")) -> (element=w367:refnum<vi>)
        n249 = property class="VI"(reference=w367) -> (reference out=w362:refnum<vi>, "Exec.State"=w361:T11)  [unwired: 1 in, 1 out]
        n250 = case shown="\"Bad\", 默认" w361 {
          tunnel: [w368 w370] -> w364
          tunnel: w362 -> [w368 w369]
          frame "Bad", Default {
          }
          frame "Idle" {
            n251 = invoke class="VI" method="Run VI"(reference=w369, "Wait until done"=FALSE ("结束前等待"), "Auto Dispose Ref"=FALSE ("自动销毁引用")) -> (reference out=w370:refnum<vi>)  [unwired: 2 in, 4 out]
          }
        }
        n252 = invoke on="探头校准子面板" class="SubPnl" method="Remove VI"() -> (error out=w363:errorcluster)  [unwired: 3 in, 2 out]
        n253 = invoke on="探头校准子面板" class="SubPnl" method="Insert VI"(error in=w363, "VI Ref"=w364) -> ()  [unwired: 2 in, 4 out]
      }
      event "pH校准": Value Change {
        n254 = event-data() -> ()  [unwired: 1 in, 6 out]
        n255 = Index Array(array=w378, index=5 ("索引")) -> (element=w379:refnum<vi>)
        n256 = property class="VI"(reference=w379) -> (reference out=w374:refnum<vi>, "Exec.State"=w373:T11)  [unwired: 1 in, 1 out]
        n257 = case shown="\"Bad\", 默认" w373 {
          tunnel: w374 -> [w380 w384]
          tunnel: [w380 w381] -> w376
          frame "Bad", Default {
          }
          frame "Idle" {
            n258 = invoke class="VI" method="Run VI"(reference=w384, "Wait until done"=FALSE ("结束前等待"), "Auto Dispose Ref"=FALSE ("自动销毁引用")) -> (reference out=w381:refnum<vi>)  [unwired: 2 in, 4 out]
          }
        }
        n259 = invoke on="探头校准子面板" class="SubPnl" method="Remove VI"() -> (error out=w375:errorcluster)  [unwired: 3 in, 2 out]
        n260 = invoke on="探头校准子面板" class="SubPnl" method="Insert VI"(error in=w375, "VI Ref"=w376) -> ()  [unwired: 2 in, 4 out]
      }
      event "电导率校准": Value Change {
        n261 = event-data() -> ()  [unwired: 1 in, 6 out]
        n262 = Index Array(array=w390, index=6 ("索引")) -> (element=w391:refnum<vi>)
        n263 = property class="VI"(reference=w391) -> (reference out=w386:refnum<vi>, "Exec.State"=w385:T11)  [unwired: 1 in, 1 out]
        n264 = case shown="\"Bad\", 默认" w385 {
          tunnel: [w392 w394] -> w388
          tunnel: w386 -> [w392 w393]
          frame "Bad", Default {
          }
          frame "Idle" {
            n265 = invoke class="VI" method="Run VI"(reference=w393, "Wait until done"=FALSE ("结束前等待"), "Auto Dispose Ref"=FALSE ("自动销毁引用")) -> (reference out=w394:refnum<vi>)  [unwired: 2 in, 4 out]
          }
        }
        n266 = invoke on="探头校准子面板" class="SubPnl" method="Remove VI"() -> (error out=w387:errorcluster)  [unwired: 3 in, 2 out]
        n267 = invoke on="探头校准子面板" class="SubPnl" method="Insert VI"(error in=w387, "VI Ref"=w388) -> ()  [unwired: 2 in, 4 out]
      }
      event "溶解氧校准": Value Change {
        n268 = event-data() -> ()  [unwired: 1 in, 6 out]
        n269 = Index Array(array=w402, index=7 ("索引")) -> (element=w403:refnum<vi>)
        n270 = property class="VI"(reference=w403) -> (reference out=w398:refnum<vi>, "Exec.State"=w397:T11)  [unwired: 1 in, 1 out]
        n271 = case shown="\"Bad\", 默认" w397 {
          tunnel: [w404 w406] -> w400
          tunnel: w398 -> [w404 w405]
          frame "Bad", Default {
          }
          frame "Idle" {
            n272 = invoke class="VI" method="Run VI"(reference=w405, "Wait until done"=FALSE ("结束前等待"), "Auto Dispose Ref"=FALSE ("自动销毁引用")) -> (reference out=w406:refnum<vi>)  [unwired: 2 in, 4 out]
          }
        }
        n273 = invoke on="探头校准子面板" class="SubPnl" method="Remove VI"() -> (error out=w399:errorcluster)  [unwired: 3 in, 2 out]
        n274 = invoke on="探头校准子面板" class="SubPnl" method="Insert VI"(error in=w399, "VI Ref"=w400) -> ()  [unwired: 2 in, 4 out]
      }
      event "浊度校准": Value Change {
        n275 = event-data() -> ()  [unwired: 1 in, 6 out]
        n276 = Index Array(array=w414, index=8 ("索引")) -> (element=w415:refnum<vi>)
        n277 = property class="VI"(reference=w415) -> (reference out=w410:refnum<vi>, "Exec.State"=w409:T11)  [unwired: 1 in, 1 out]
        n278 = case shown="\"Bad\", 默认" w409 {
          tunnel: [w416 w418] -> w412
          tunnel: w410 -> [w416 w417]
          frame "Bad", Default {
          }
          frame "Idle" {
            n279 = invoke class="VI" method="Run VI"(reference=w417, "Wait until done"=FALSE ("结束前等待"), "Auto Dispose Ref"=FALSE ("自动销毁引用")) -> (reference out=w418:refnum<vi>)  [unwired: 2 in, 4 out]
          }
        }
        n280 = invoke on="探头校准子面板" class="SubPnl" method="Remove VI"() -> (error out=w411:errorcluster)  [unwired: 3 in, 2 out]
        n281 = invoke on="探头校准子面板" class="SubPnl" method="Insert VI"(error in=w411, "VI Ref"=w412) -> ()  [unwired: 2 in, 4 out]
      }
      event "叶绿素a校准": Value Change {
        n282 = event-data() -> ()  [unwired: 1 in, 6 out]
        n283 = Index Array(array=w426, index=9 ("索引")) -> (element=w427:refnum<vi>)
        n284 = property class="VI"(reference=w427) -> (reference out=w422:refnum<vi>, "Exec.State"=w421:T11)  [unwired: 1 in, 1 out]
        n285 = case shown="\"Bad\", 默认" w421 {
          tunnel: [w428 w430] -> w424
          tunnel: w422 -> [w428 w429]
          frame "Bad", Default {
          }
          frame "Idle" {
            n286 = invoke class="VI" method="Run VI"(reference=w429, "Wait until done"=FALSE ("结束前等待"), "Auto Dispose Ref"=FALSE ("自动销毁引用")) -> (reference out=w430:refnum<vi>)  [unwired: 2 in, 4 out]
          }
        }
        n287 = invoke on="探头校准子面板" class="SubPnl" method="Remove VI"() -> (error out=w423:errorcluster)  [unwired: 3 in, 2 out]
        n288 = invoke on="探头校准子面板" class="SubPnl" method="Insert VI"(error in=w423, "VI Ref"=w424) -> ()  [unwired: 2 in, 4 out]
      }
    }
  }
